vi "Control Box.vi"(0 "detection controls":T2, 7 "Sorting parameters":T4, 9 "Array":dbl[][](array[numeric]), 11 "Function generator":T6) -> (4 "detection controls":T1, 8 "Sorting parameters":T3, 10 "Array 2":cluster{"[0]":i32, "[1]":i32, "[2]":i32}[](array[cluster]), 15 "Function generator":T5)   [LabVIEW 2009]
panel:
  out "unsigned 32bit integer":u32
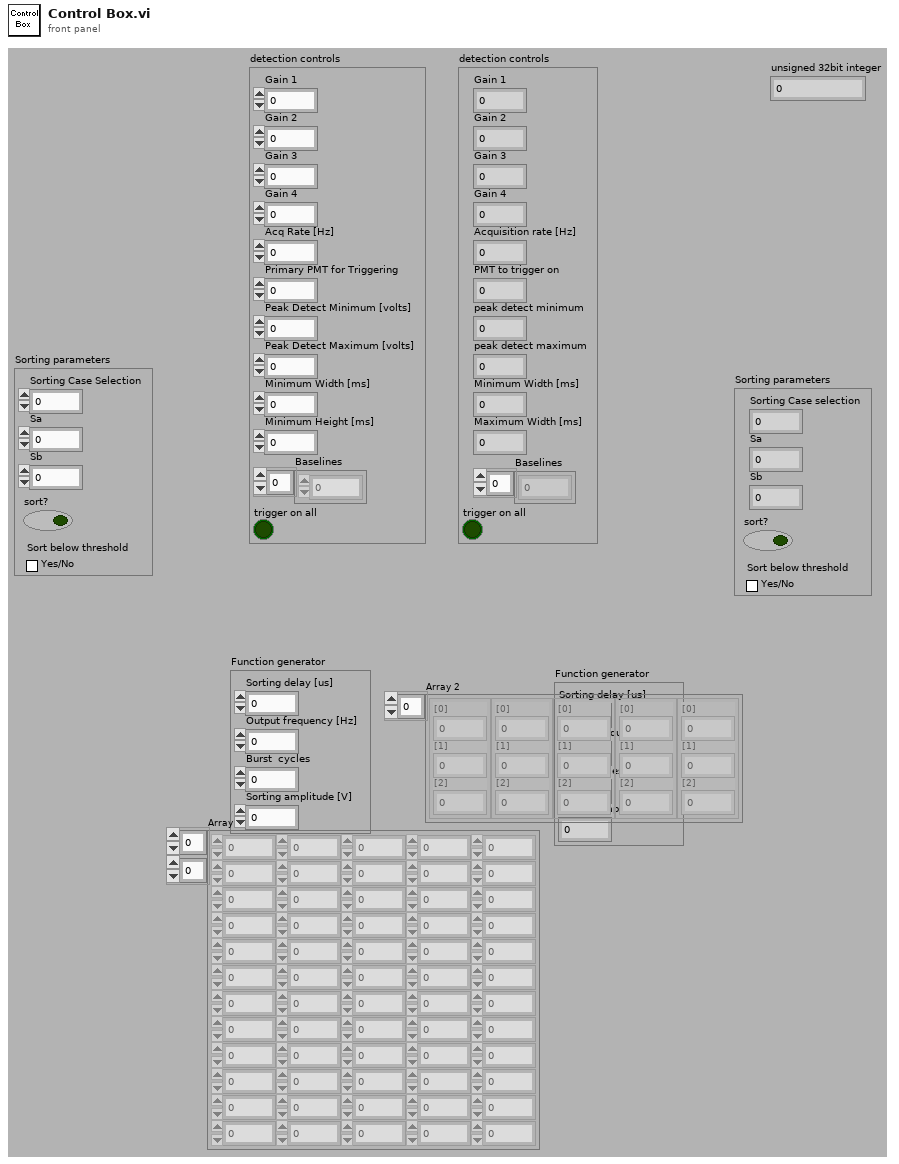
[diagram p1: front panel]
types:
  T1 = cluster{"Gain 1":i16, "Gain 2":i16, "Gain 3":i16, "Gain 4":i16, "Acquisition rate [Hz]":u32, "PMT to trigger on":u8, "peak detect minimum":i16, "peak detect maximum":i16, "Minimum Width [ms]":i16, "Maximum Width [ms]":i16, "Baselines":i16[], "trigger on all":bool}
  T2 = cluster{"Gain 1":sgl, "Gain 2":sgl, "Gain 3":sgl, "Gain 4":sgl, "Acq Rate [Hz]":dbl, "Primary PMT for Triggering":u8, "Peak Detect Minimum [volts]":dbl, "Peak Detect Maximum [volts]":dbl, "Minimum Width [ms]":dbl, "Minimum Height [ms]":dbl, "Baselines":dbl[], "trigger on all":bool}
  T3 = cluster{"Sorting Case selection":i8, "Sa":i8, "Sb":i8, "sort?":bool, "Sort below threshold":bool}
  T4 = cluster{"Sorting Case Selection":i8, "Sa":i8, "Sb":i8, "sort?":bool, "Sort below threshold":bool}
  T5 = cluster{"Sorting delay [us]":u32, "Output frequency [Hz]":u32, "Burst  cycles":i32, "Sorting amplitude [V]":i16}
  T6 = cluster{"Sorting delay [us]":u32, "Output frequency [Hz]":u32, "Burst  cycles":i32, "Sorting amplitude [V]":dbl}
  T7 = cluster{"Gain 1":i16, "Gain 2":i16, "Gain 3":i16, "Gain 4":i16, "Acquisition rate [Hz]":u32, "PMT to trigger on":u8, "peak detect treshold":i16, "peak detect maximum":i16, "Minimum Width [ms]":i16, "Maximum Width [ms]":i16, "Baselines":i16[], "trigger on all":bool}
  T8 = cluster{"Sorting delay [us]":u32, u32, "Burst  cycles":i32, i16}
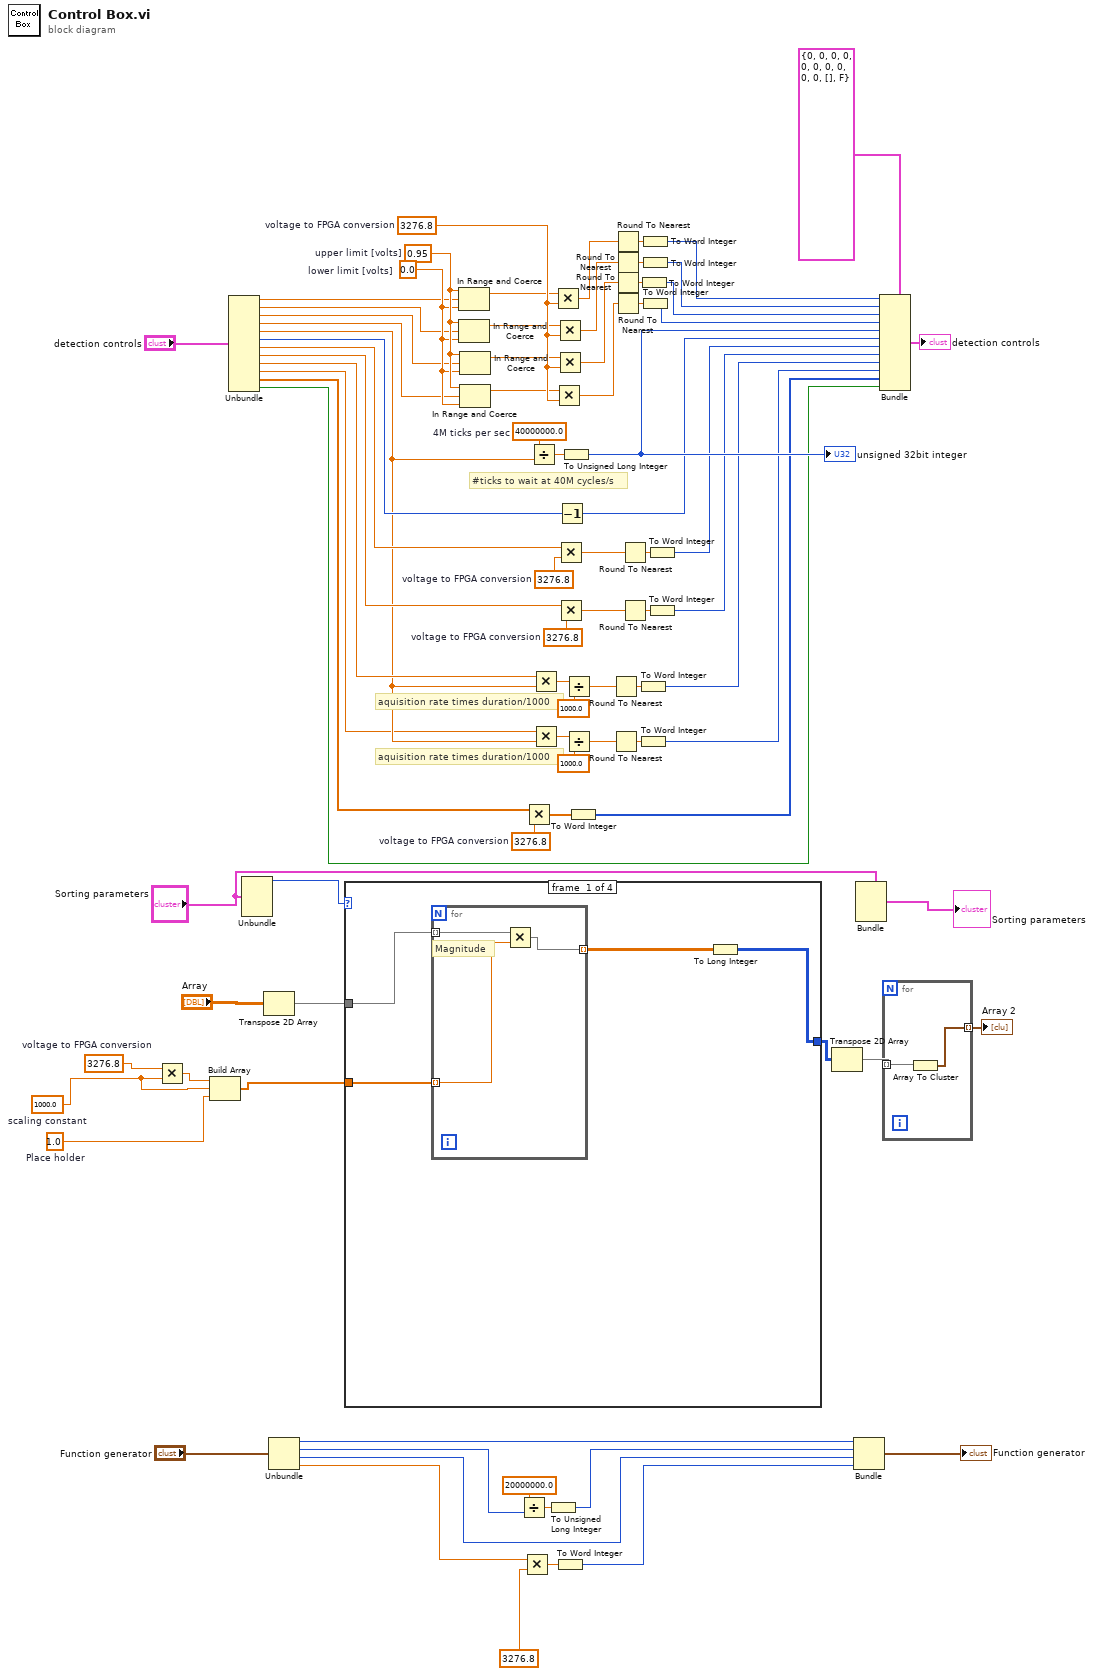
[diagram p0: block diagram]
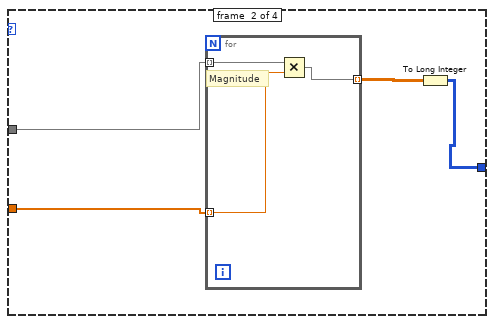
[diagram p2: hidden frame]
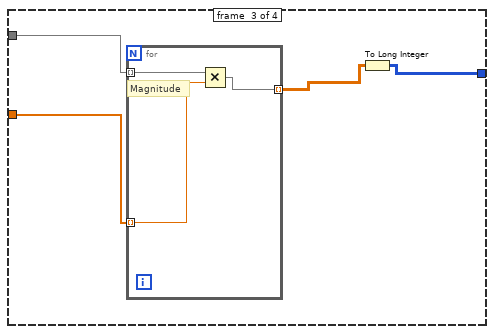
[diagram p3: hidden frame]
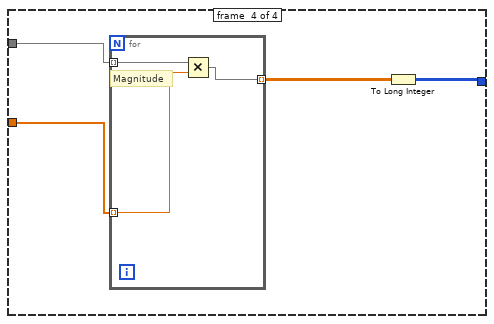
[diagram p4: hidden frame]
diagram:
  w5 = 1.0  # Place holder
  w6 = 1000.0  # scaling constant
  w8 = 3276.8  # voltage to FPGA conversion
  w29 = 3276.8  # voltage to FPGA conversion
  w75 = 3276.8  # voltage to FPGA conversion
  w28 = 3276.8  # voltage to FPGA conversion
  w83 = 40000000.0  # 4M ticks per sec
  w82 = 0.95  # upper limit [volts]
  w81 = 3276.8  # voltage to FPGA conversion
  w76 = 0.0  # lower limit [volts]
  # "aquisition rate times duration/1000"
  # "aquisition rate times duration/1000"
  # "#ticks to wait at 40M cycles/s"
  n1 = Multiply(x=w8, y=w6) -> (x*y=w7:dbl)
  n2 = Build Array(w7, w6, w5) -> (w4:dbl[])
  n3 = Unbundle("detection controls") -> ("Gain 1"=w37:sgl, "Gain 2"=w36:sgl, "Gain 3"=w35:sgl, "Gain 4"=w34:sgl, "Acq Rate [Hz]"=w21:dbl, "Primary PMT for Triggering"=w33:u8, "Peak Detect Minimum [volts]"=w32:dbl, "Peak Detect Maximum [volts]"=w23:dbl, "Minimum Width [ms]"=w22:dbl, "Minimum Height [ms]"=w20:dbl, "Baselines"=w19:dbl[], "trigger on all"=w13:bool)
  n4 = Unbundle("Sorting parameters") -> ("Sorting Case Selection"=w11:i8)  [unwired: 4 out]
  n5 = Transpose 2D Array(2D array="Array") -> (transposed array=w9:dbl[][])
  n6 = Unbundle("Function generator") -> ("Sorting delay [us]"=w62:u32, "Output frequency [Hz]"=w64:u32, "Burst  cycles"=w60:i32, "Sorting amplitude [V]"=w63:dbl)
  n7 = case shown="0, Default" w11 {
    tunnel: w9 -> [w88 w94 w102 w108]
    tunnel: w4 -> [w87 w93 w101 w107]
    tunnel: [w85 w92 w99 w106] -> w2
    frame #0 {
      n8 = for {
        tunnel: w88 -> [w91] mode=indexing
        tunnel: w87 -> [w90] mode=indexing
        tunnel: [w89] -> w86 mode=indexing
        # "Magnitude"
        n9 = Multiply(x=w91, y=w90) -> (x*y=w89:dbl[])
      }
      n10 = To Long Integer(number=w86) -> (32bit integer=w85:i32[][])
    }
    frame #1 {
      n11 = for {
        tunnel: w94 -> [w98] mode=indexing
        tunnel: w93 -> [w97] mode=indexing
        tunnel: [w96] -> w95 mode=indexing
        # "Magnitude"
        n12 = Multiply(x=w98, y=w97) -> (x*y=w96:dbl[])
      }
      n13 = To Long Integer(number=w95) -> (32bit integer=w92:i32[][])
    }
    frame #2 {
      n14 = for {
        tunnel: w102 -> [w105] mode=indexing
        tunnel: w101 -> [w104] mode=indexing
        tunnel: [w103] -> w100 mode=indexing
        # "Magnitude"
        n15 = Multiply(x=w105, y=w104) -> (x*y=w103:dbl[])
      }
      n16 = To Long Integer(number=w100) -> (32bit integer=w99:i32[][])
    }
    frame #3 {
      n17 = for {
        tunnel: w108 -> [w112] mode=indexing
        tunnel: w107 -> [w111] mode=indexing
        tunnel: [w110] -> w109 mode=indexing
        # "Magnitude"
        n18 = Multiply(x=w112, y=w111) -> (x*y=w110:dbl[])
      }
      n19 = To Long Integer(number=w109) -> (32bit integer=w106:i32[][])
    }
  }
  n20 = In Range and Coerce(upper limit=w82, x=w37, lower limit=w76) -> (coerced(x)=w77:dbl)  [unwired: 1 out]
  n21 = In Range and Coerce(upper limit=w82, x=w36, lower limit=w76) -> (coerced(x)=w80:dbl)  [unwired: 1 out]
  n22 = In Range and Coerce(upper limit=w82, x=w35, lower limit=w76) -> (coerced(x)=w79:dbl)  [unwired: 1 out]
  n23 = In Range and Coerce(upper limit=w82, x=w34, lower limit=w76) -> (coerced(x)=w78:dbl)  [unwired: 1 out]
  n24 = Divide(x=20000000.0 ("y"), y=w64) -> (x/y=w66:dbl)
  n25 = Multiply(x=w63, y=3276.8) -> (x*y=w67:dbl)
  n26 = Multiply(x=w19, y=w75) -> (x*y=w70:dbl[])
  n27 = Divide(x=w83, y=w21) -> (x/y=w84:dbl)
  n28 = Multiply(x=w22, y=w21) -> (x*y=w73:dbl)
  n29 = Multiply(x=w20, y=w21) -> (x*y=w24:dbl)
  n30 = To Unsigned Long Integer(number=w66) -> (unsigned 32bit integer=w61:u32)
  n31 = Multiply(x=w77, y=w81) -> (x*y=w56:dbl)
  n32 = Multiply(x=w78, y=w81) -> (x*y=w47:dbl)
  n33 = Multiply(x=w80, y=w81) -> (x*y=w51:dbl)
  n34 = Multiply(x=w79, y=w81) -> (x*y=w49:dbl)
  n35 = To Word Integer(number=w67) -> (16bit integer=w59:i16)
  n36 = Multiply(x=w32, y=w28) -> (x*y=w43:dbl)
  n37 = Multiply(x=w23, y=w29) -> (x*y=w31:dbl)
  n38 = Decrement(x=w33) -> (x-1=w71:u8)
  n39 = To Unsigned Long Integer(number=w84) -> (unsigned 32bit integer=w74:u32)
  "unsigned 32bit integer" <- w74
  n40 = Divide(x=w73, y=1000.0) -> (x/y=w41:dbl)
  n41 = Divide(x=w24, y=1000.0) -> (x/y=w27:dbl)
  n42 = To Word Integer(number=w70) -> (16bit integer=w14:i16[])
  n43 = Round To Nearest(number=w41) -> (nearest integer value=w45:dbl)
  n44 = Round To Nearest(number=w27) -> (nearest integer value=w26:dbl)
  n45 = Round To Nearest(number=w56) -> (nearest integer value=w57:dbl)
  n46 = Round To Nearest(number=w51) -> (nearest integer value=w54:dbl)
  n47 = Round To Nearest(number=w49) -> (nearest integer value=w53:dbl)
  n48 = Round To Nearest(number=w47) -> (nearest integer value=w52:dbl)
  n49 = Round To Nearest(number=w43) -> (nearest integer value=w44:dbl)
  n50 = Round To Nearest(number=w31) -> (nearest integer value=w30:dbl)
  n51 = To Word Integer(number=w45) -> (16bit integer=w16:i16)
  n52 = To Word Integer(number=w26) -> (16bit integer=w15:i16)
  n53 = To Word Integer(number=w53) -> (16bit integer=w48:i16)
  n54 = To Word Integer(number=w57) -> (16bit integer=w55:i16)
  n55 = To Word Integer(number=w54) -> (16bit integer=w50:i16)
  n56 = To Word Integer(number=w52) -> (16bit integer=w46:i16)
  n57 = To Word Integer(number=w44) -> (16bit integer=w42:i16)
  n58 = To Word Integer(number=w30) -> (16bit integer=w17:i16)
  n59 = Transpose 2D Array(2D array=w2) -> (transposed array=w3:i32[][])
  n60 = Bundle("Sorting delay [us]"=w62, w61, "Burst  cycles"=w60, w59) -> (→"Function generator":T8)  [unwired: 1 in]
  n61 = Bundle(cluster="Sorting parameters") -> (→"Sorting parameters":T4)  [unwired: 5 in]
  n62 = Bundle(cluster=T7 {"Gain 1"=0, "Gain 2"=0, "Gain 3"=0, "Gain 4"=0, "Acquisition rate [Hz]"=0, "PMT to trigger on"=0, "peak detect treshold"=0, "peak detect maximum"=0, "Minimum Width [ms]"=0, "Maximum Width [ms]"=0, "Baselines"=[], "trigger on all"=FALSE} ("FPGA Parameters 2"), "Gain 1"=w55, "Gain 2"=w50, "Gain 3"=w48, "Gain 4"=w46, "Acquisition rate [Hz]"=w74, "PMT to trigger on"=w71, "peak detect treshold"=w42, "peak detect maximum"=w17, "Minimum Width [ms]"=w16, "Maximum Width [ms]"=w15, "Baselines"=w14, "trigger on all"=w13) -> (→"detection controls":T7)
  n63 = for {
    tunnel: [w113] -> w1 mode=indexing
    tunnel: w3 -> [w114] mode=indexing
    n64 = Array To Cluster(array=w114) -> (cluster=w113:cluster{"[0]":i32, "[1]":i32, "[2]":i32})
  }
  "Array 2" <- w1
